vi "AlGaInPAs_prep_run_cont_dil_v15.vi"(2 "Debug Mode":bool, 3 "Elapsed Time(s)":dbl, 4 "State":enum16{"Edit", "Start", "Run", "End", "Idle"}(ring), 5 "Argument List In":string[](array[string])) -> (0 "Status Out":string, 1 "Argument List Out":string[](array[string]))   [LabVIEW 2011]
panel:
  out "Ga calculated var":u16(ring)=1 items=["Ga flow", "MFC1", "MFC2", "MFC3"]
  out "GAMFC3 var":dbl=100.0 caption="R3 (0-1000 sscm)" format="%.1f"
  out "GAMFC2 var":dbl=10.0 caption="R2 (0-100 sscm)" format="%.2f"
  out "GAMFC1 var":dbl=1.0 caption="R1 (0-10 sscm)" format="%.2f"
  out "Ga Flow var":dbl=1.0 caption="Ga Flow (0-10 sscm)" format="%.4f"
  out "Prep-In var":bool
  out "Prep-Ga var":bool
  out "Prep-Al var":bool
  out "Prep-P var":bool
  out "Prep-As var":bool
  out "prep_done":bool
  out "run started":bool
  out "first":bool=TRUE
  out "total time":dbl
  out "is OK?":bool
  out "AsH3?":bool
  out "PH3?":bool
  out "In?":bool
  out "Ga?":bool
  out "Al?":bool
  in  "Prep As":bool caption="Pre-run"
  in  "Prep P":bool caption="Pre-run"
  in  "Prep In":bool caption="Pre-run"
  in  "prep_time":dbl caption="pre-run time (s)"
  in  "Prep Al":bool caption="Pre-run"
  in  "Run As":bool caption="Run"
  in  "AsH3 Flow":dbl caption="AsH3 Flow (0-10 sccm)" format="%.2f"
  in  "P Flow":dbl caption="P Flow (0-100 sccm)" format="%.2f"
  in  "Run P":bool caption="Run"
  in  "In Flow":dbl caption="In Flow (0-100 sscm)" format="%.2f"
  in  "Run In":bool caption="Run"
  in  "Run Al":bool caption="Run"
  in  "Al Flow":dbl caption="Al Flow (0-100 sscm)" format="%.2f"
  in  "Cancel":bool
  in  "OK":bool
  out "tTotal(s) 2":dbl
  in  "Ga Tab Control":enum32{"Page 1", "Page 2", "Page 3"}(tab)
  in  "Ga Dilution":bool caption="Dilute"
  in  "Run Ga":bool caption="Run"
  in  "Prep Ga":bool caption="Pre-run"
  out "Ga Flow val":dbl=1.0 caption="Ga Flow (0-10 sscm)" format="%.4f"
  in  "Ga Flow set":dbl=1.0 caption="Ga Flow (0-10 sscm)" format="%.4f"
  out "GAMFC1 val":dbl=1.0 caption="R1 (0-10 sscm)" format="%.2f"
  out "GAMFC3 val":dbl=100.0 caption="R3 (0-1000 sscm)" format="%.1f"
  out "GAMFC2 val":dbl=10.0 caption="R2 (0-100 sscm)" format="%.2f"
  in  "GAMFC1 set":dbl=1.0 caption="R1 (0-10 sscm)" format="%.2f"
  in  "GAMFC2 set":dbl=10.0 caption="R2 (0-100 sscm)" format="%.2f"
  in  "GAMFC3 set":dbl=100.0 caption="R3 (0-1000 sscm)" format="%.1f"
  in  "Ga calculated":u16(ring)=1 items=["Ga flow", "MFC1", "MFC2", "MFC3"]
  # "Add pre-run time to run time in editor."
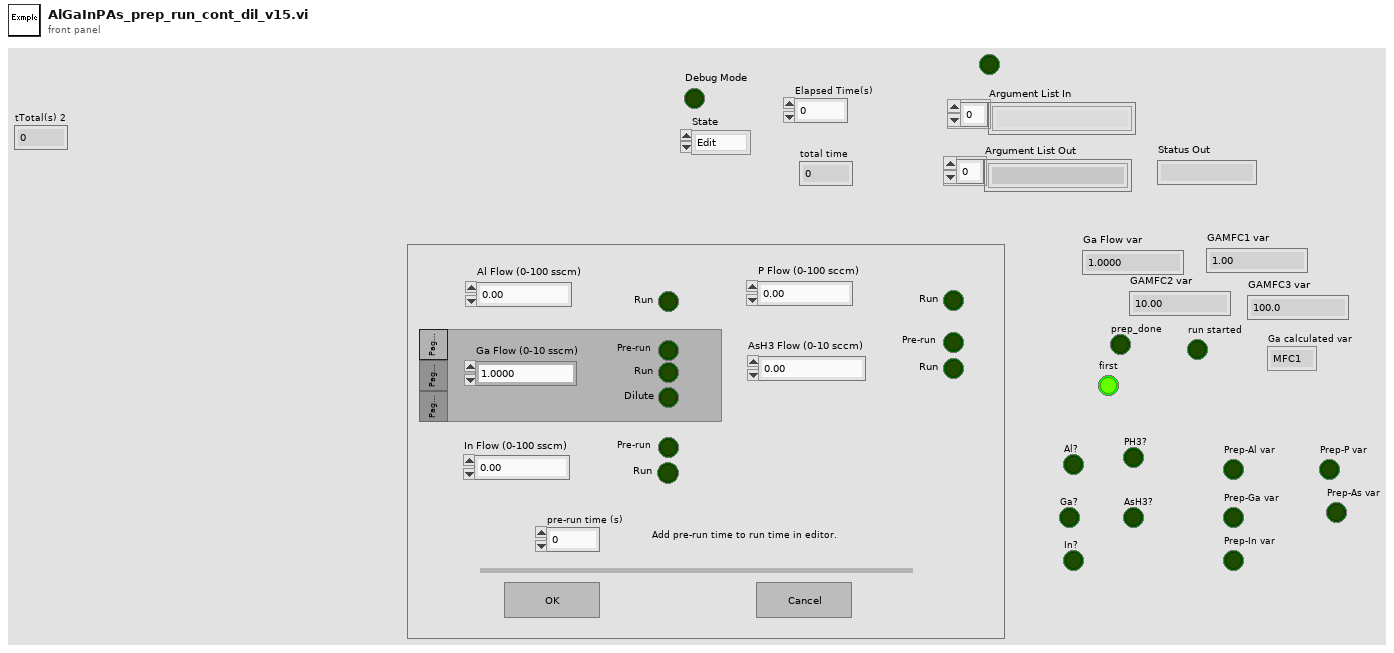
[diagram p1: front panel]
types:
  T1 = enum16{"Discrete", "Continuous", "Instantaneous", "Finite"}
  T2 = enum32{"Invalid", "Default", "Floating", "Floating/Auto-Hide", "Modal"}
  T3 = cluster{"Visible":bool, "Visible":bool, "Visible":bool, "Visible":bool, "Visible":bool, "Visible":bool, "Visible":bool, "Visible":bool}
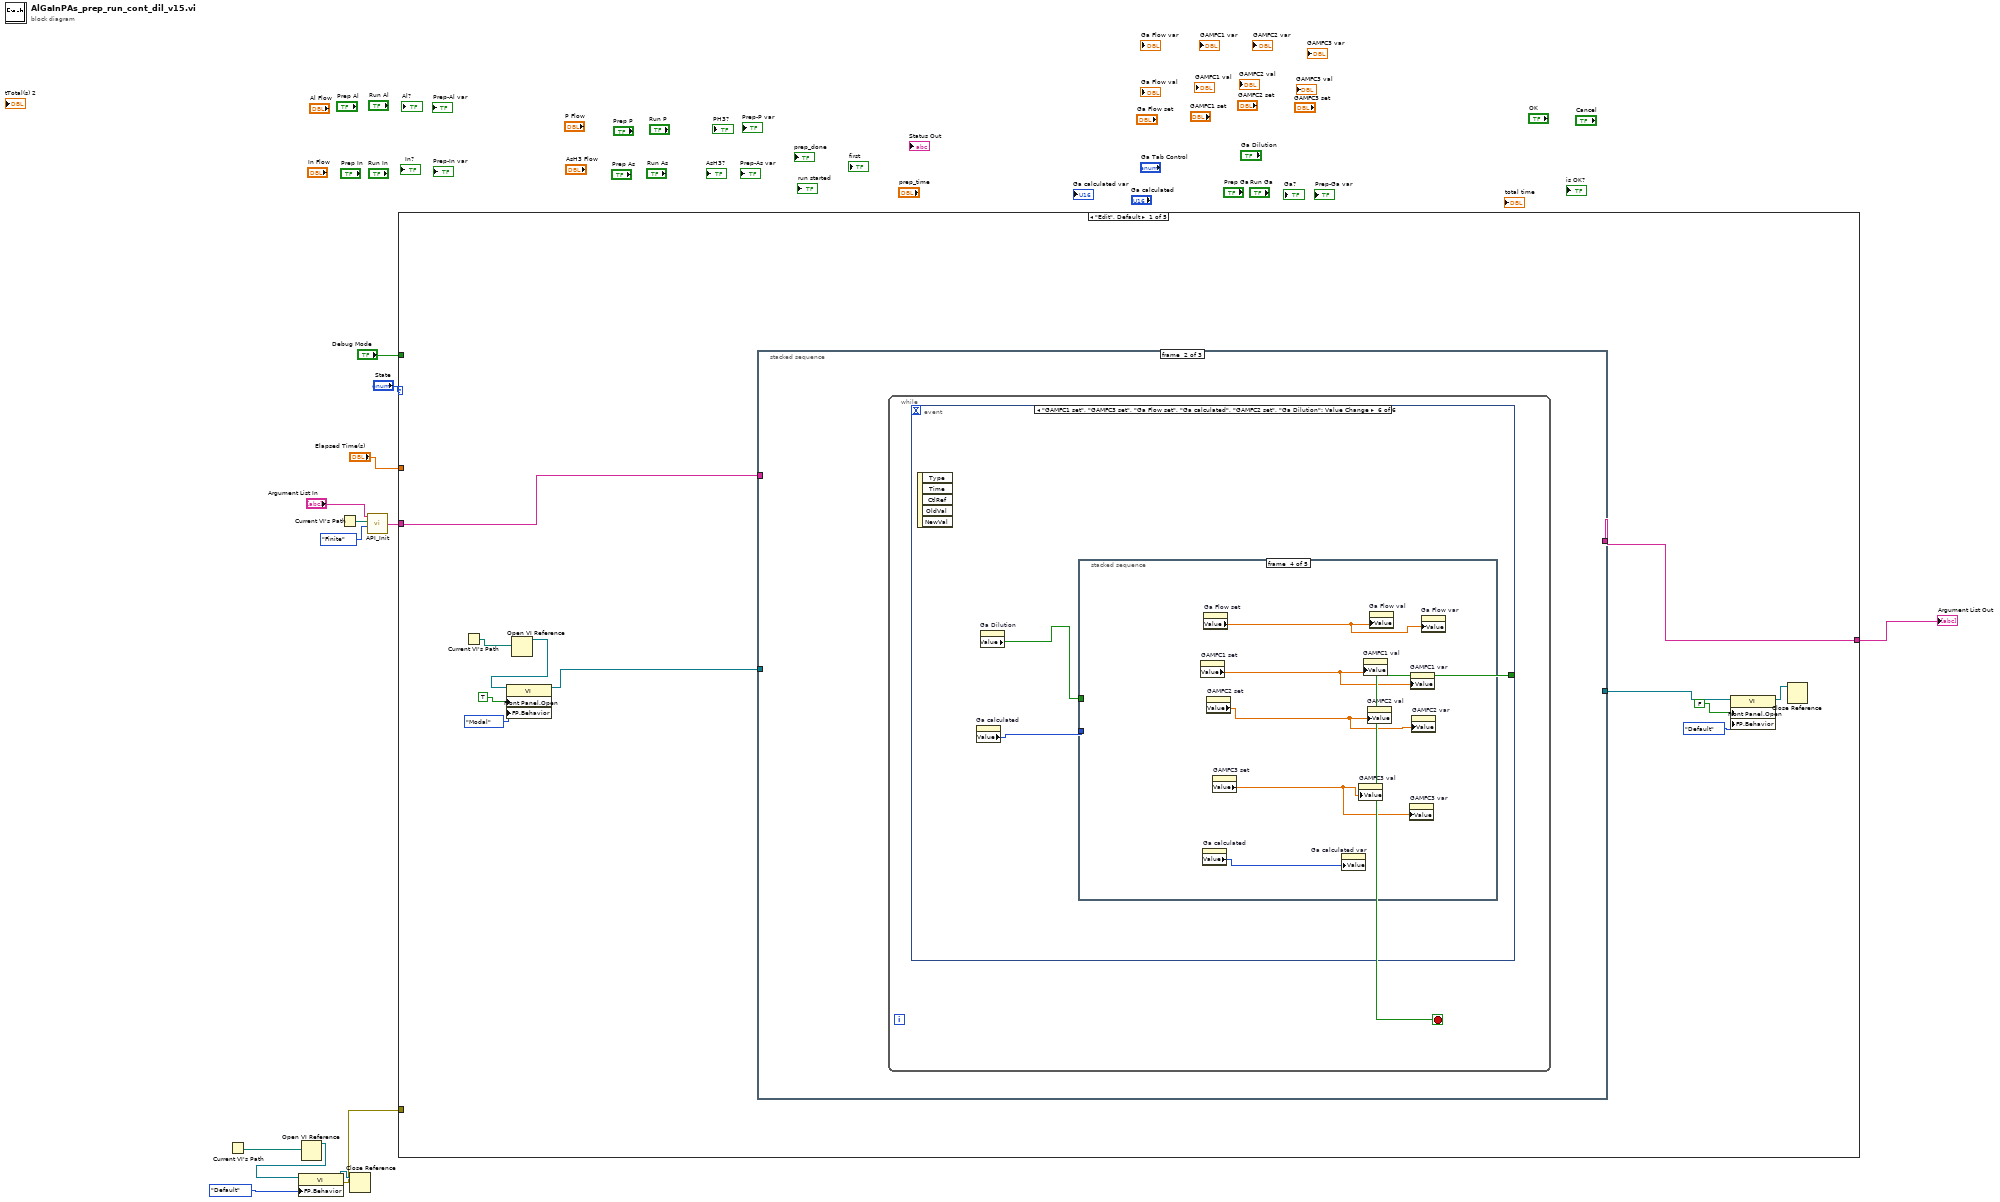
[diagram p0: block diagram]
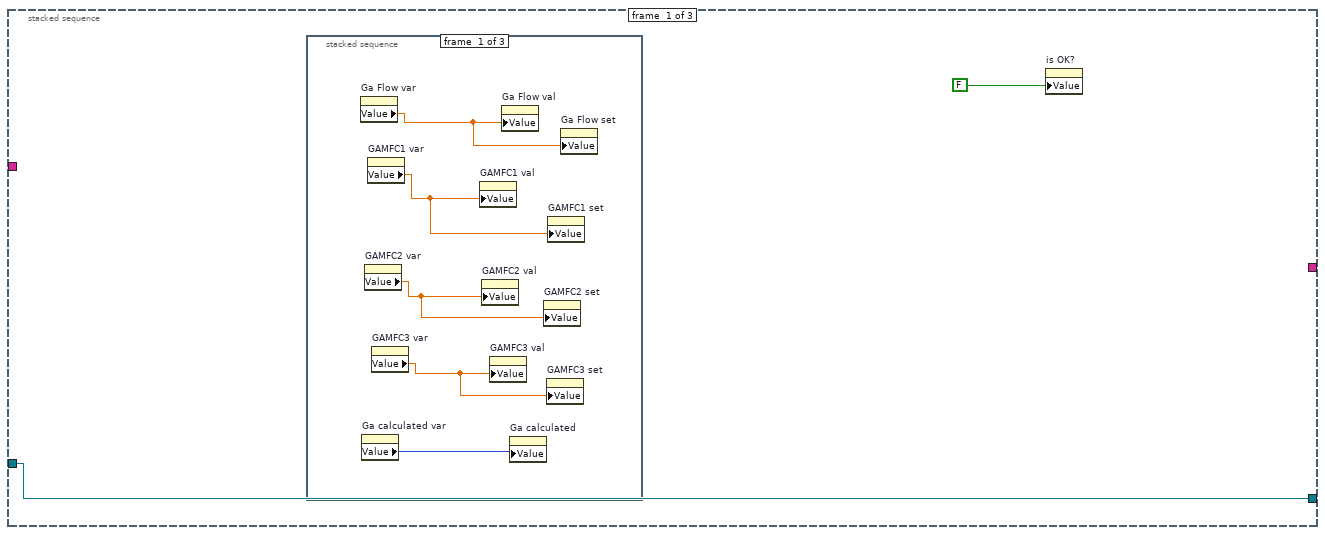
[diagram p2: hidden frame]
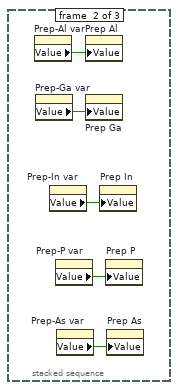
[diagram p3: hidden frame]
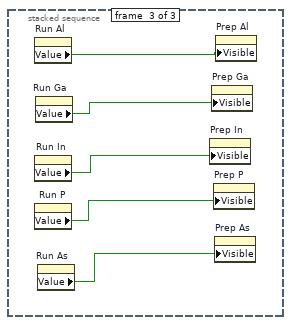
[diagram p4: hidden frame]
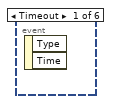
[diagram p5: hidden frame]
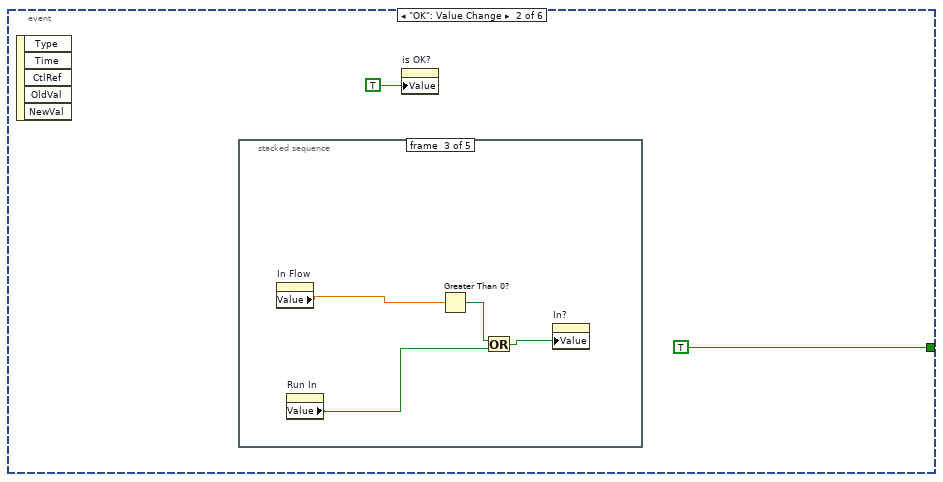
[diagram p6: hidden frame]
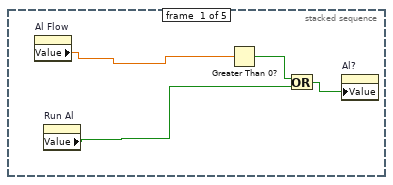
[diagram p7: hidden frame]
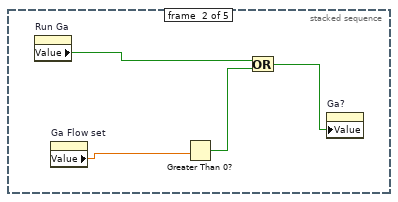
[diagram p8: hidden frame]
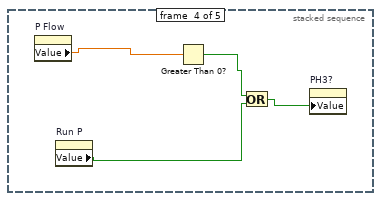
[diagram p9: hidden frame]
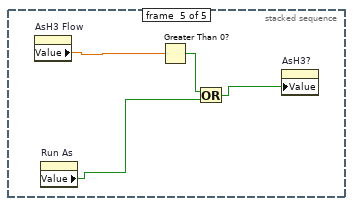
[diagram p10: hidden frame]
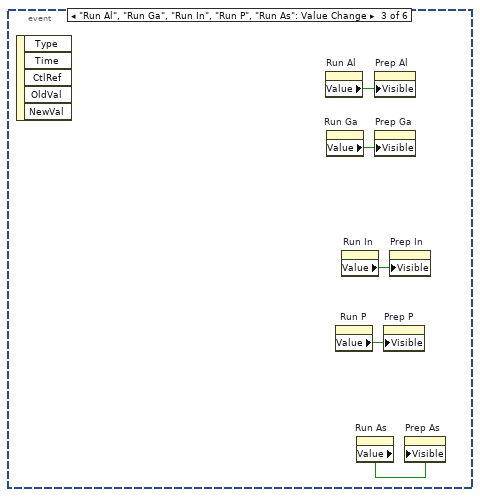
[diagram p11: hidden frame]
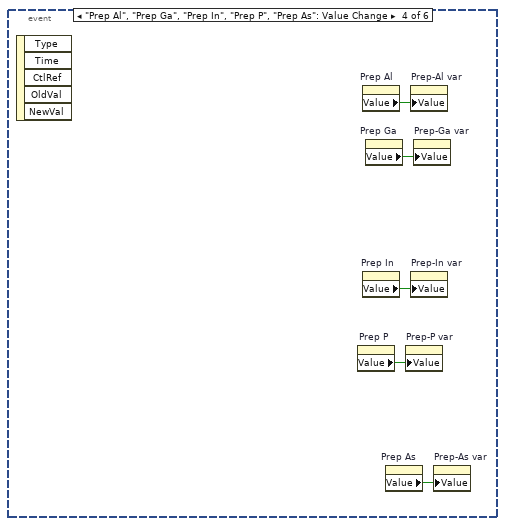
[diagram p12: hidden frame]
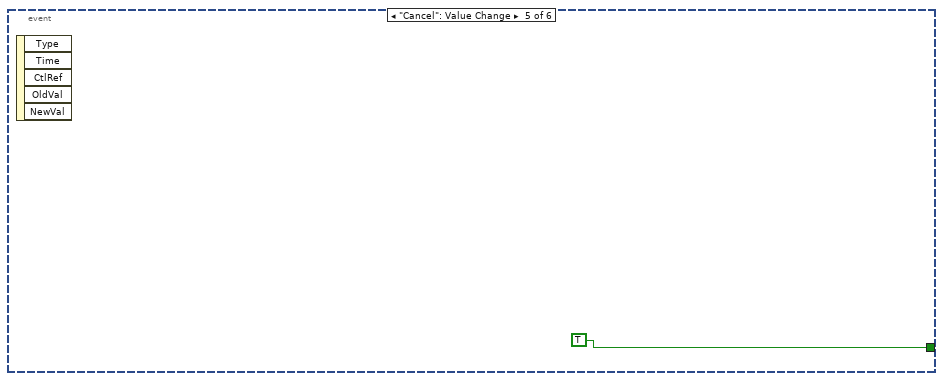
[diagram p13: hidden frame]
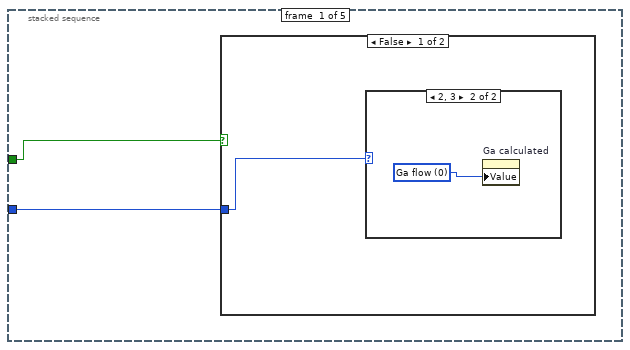
[diagram p14: hidden frame]
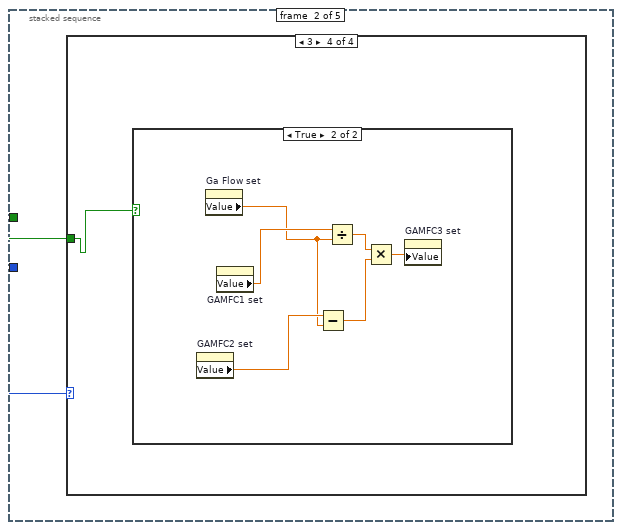
[diagram p17: hidden frame]
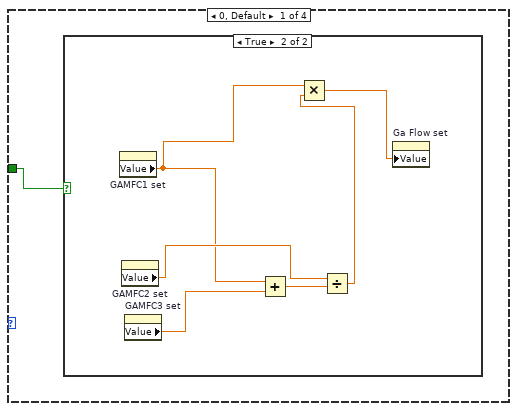
[diagram p18: hidden frame]
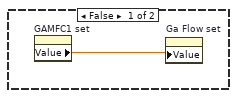
[diagram p19: hidden frame]
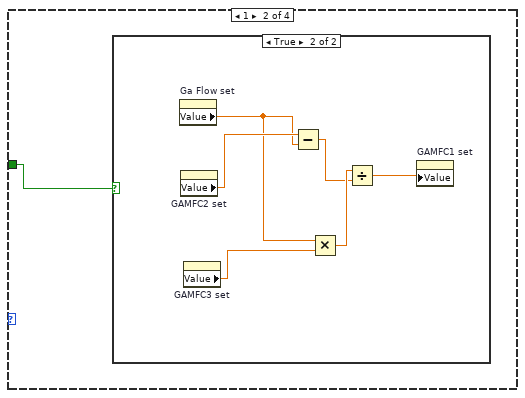
[diagram p20: hidden frame]
diagram:
  n1 = Current VI's Path() -> (path=w9:path)
  n2 = Open VI Reference(vi path=w9) -> (vi reference=w8:refnum<vi>)  [unwired: 1 in, 5 out]
  n3 = property class="VI"(reference=w8, "FP.Behavior"=T2."Default" ("Front Panel Window:Behavior")) -> (reference out=w6:refnum<vi>, error out=w5:errorcluster)  [unwired: 1 in]
  n4 = Current VI's Path() -> (path=w4:path)
  n5 = Close Reference(reference=w6) -> ()  [unwired: 1 in, 1 out]
  n6 = call "API_Init.vi"("API Mode"=T1."Finite", "VI Path"=w4, "Argument List In"="Argument List In") -> ("Argument List Out"=w1:string[])  [unwired: 1 in]
  n7 = case shown="\"Edit\", Default" "State" {
    tunnel: "Debug Mode" -> [_ w175 w229 _ _]
    tunnel: "Elapsed Time(s)" -> [_ _ w231 _ _]
    tunnel: w1 -> [w15 w177 w228 w346 w347]
    tunnel: [w14 w176 w230 w346 w347] -> w10
    tunnel: w5 -> [_ _ _ _ _]
    frame "Edit", Default {
      n8 = Current VI's Path() -> (path=w20:path)
      n9 = Open VI Reference(vi path=w20) -> (vi reference=w19:refnum<vi>)  [unwired: 1 in, 5 out]
      n10 = property class="VI"(reference=w19, "Front Panel.Open"=TRUE ("Front Panel Window:Open"), "FP.Behavior"=T2."Modal" ("Front Panel Window:Behavior")) -> (reference out=w18:refnum<vi>)  [unwired: 1 in, 1 out]
      n11 = stacked-sequence {
        tunnel: w15 -> [_ _ w170]
        tunnel: w18 -> [w26 _ _]
        tunnel: [w26 _ _] -> w22
        tunnel: [_ _ w168] -> w14
        frame #0 {
          n12 = stacked-sequence {
            frame #0 {
              n13 = property on="Ga Flow var" class="DigNum (strict)"() -> ("Value"=w31:dbl)  [unwired: 2 in, 2 out]
              n14 = property on="Ga calculated var" class="Ring (strict)"() -> ("Value"=w27:u16)  [unwired: 2 in, 2 out]
              n15 = property on="GAMFC2 var" class="DigNum (strict)"() -> ("Value"=w29:dbl)  [unwired: 2 in, 2 out]
              n16 = property on="GAMFC1 var" class="DigNum (strict)"() -> ("Value"=w28:dbl)  [unwired: 2 in, 2 out]
              n17 = property on="GAMFC3 var" class="DigNum (strict)"() -> ("Value"=w30:dbl)  [unwired: 2 in, 2 out]
              n18 = property on="GAMFC1 val" class="DigNum (strict)"("Value"=w28) -> ()  [unwired: 2 in, 2 out]
              n19 = property on="GAMFC2 val" class="DigNum (strict)"("Value"=w29) -> ()  [unwired: 2 in, 2 out]
              n20 = property on="GAMFC3 val" class="DigNum (strict)"("Value"=w30) -> ()  [unwired: 2 in, 2 out]
              n21 = property on="Ga Flow val" class="DigNum (strict)"("Value"=w31) -> ()  [unwired: 2 in, 2 out]
              n22 = property on="Ga calculated" class="Ring (strict)"("Value"=w27) -> ()  [unwired: 2 in, 2 out]
              n23 = property on="GAMFC2 set" class="DigNum (strict)"("Value"=w29) -> ()  [unwired: 2 in, 2 out]
              n24 = property on="GAMFC3 set" class="DigNum (strict)"("Value"=w30) -> ()  [unwired: 2 in, 2 out]
              n25 = property on="GAMFC1 set" class="DigNum (strict)"("Value"=w28) -> ()  [unwired: 2 in, 2 out]
              n26 = property on="Ga Flow set" class="DigNum (strict)"("Value"=w31) -> ()  [unwired: 2 in, 2 out]
            }
            frame #1 {
              n27 = property on="Prep-Al var" class="Bool (strict)"() -> ("Value"=w36:bool)  [unwired: 2 in, 2 out]
              n28 = property on="Prep-Ga var" class="Bool (strict)"() -> ("Value"=w35:bool)  [unwired: 2 in, 2 out]
              n29 = property on="Prep-In var" class="Bool (strict)"() -> ("Value"=w34:bool)  [unwired: 2 in, 2 out]
              n30 = property on="Prep-P var" class="Bool (strict)"() -> ("Value"=w33:bool)  [unwired: 2 in, 2 out]
              n31 = property on="Prep-As var" class="Bool (strict)"() -> ("Value"=w32:bool)  [unwired: 2 in, 2 out]
              n32 = property on="Prep Al" class="Bool (strict)"("Value"=w36) -> ()  [unwired: 2 in, 2 out]
              n33 = property on="Prep Ga" class="Bool (strict)"("Value"=w35) -> ()  [unwired: 2 in, 2 out]
              n34 = property on="Prep In" class="Bool (strict)"("Value"=w34) -> ()  [unwired: 2 in, 2 out]
              n35 = property on="Prep P" class="Bool (strict)"("Value"=w33) -> ()  [unwired: 2 in, 2 out]
              n36 = property on="Prep As" class="Bool (strict)"("Value"=w32) -> ()  [unwired: 2 in, 2 out]
            }
            frame #2 {
              n37 = property on="Run Al" class="Bool (strict)"() -> ("Value"=w41:bool)  [unwired: 2 in, 2 out]
              n38 = property on="Run In" class="Bool (strict)"() -> ("Value"=w39:bool)  [unwired: 2 in, 2 out]
              n39 = property on="Run P" class="Bool (strict)"() -> ("Value"=w38:bool)  [unwired: 2 in, 2 out]
              n40 = property on="Run Ga" class="Bool (strict)"() -> ("Value"=w40:bool)  [unwired: 2 in, 2 out]
              n41 = property on="Run As" class="Bool (strict)"() -> ("Value"=w37:bool)  [unwired: 2 in, 2 out]
              n42 = property on="Prep In" class="Bool (strict)"("Visible"=w39) -> ()  [unwired: 2 in, 2 out]
              n43 = property on="Prep Ga" class="Bool (strict)"("Visible"=w40) -> ()  [unwired: 2 in, 2 out]
              n44 = property on="Prep P" class="Bool (strict)"("Visible"=w38) -> ()  [unwired: 2 in, 2 out]
              n45 = property on="Prep As" class="Bool (strict)"("Visible"=w37) -> ()  [unwired: 2 in, 2 out]
              n46 = property on="Prep Al" class="Bool (strict)"("Visible"=w41) -> ()  [unwired: 2 in, 2 out]
            }
          }
          n47 = property on="is OK?" class="Bool (strict)"("Value"=FALSE ("is OK?")) -> ()  [unwired: 2 in, 2 out]
        }
        frame #1 {
          n48 = while {
            stop <- w42 stop-if-true
            n49 = event shown="[5] \"GAMFC1 set\", \"GAMFC3 set\", \"Ga Flow set\", \"Ga calculated\", \"GAMFC2 set\", \"Ga Dilution\": Value Change" {
              selector: _ -> [_ _ _ _ _ _]
              dyn-events: _ -> [_ _ _ _ _ _]
              timeout: _ -> [_ _ _ _ _ _]
              tunnel: [_ TRUE _ _ TRUE _] -> w42
              event Timeout {
                n50 = event-data() -> ()  [unwired: 1 in, 2 out]
              }
              event "OK": Value Change {
                n51 = event-data() -> ()  [unwired: 1 in, 5 out]
                n52 = stacked-sequence {
                  frame #0 {
                    n53 = property on="Al Flow" class="DigNum (strict)"() -> ("Value"=w47:dbl)  [unwired: 2 in, 2 out]
                    n54 = property on="Run Al" class="Bool (strict)"() -> ("Value"=w46:bool)  [unwired: 2 in, 2 out]
                    n55 = Greater Than 0?(x=w47) -> (x > 0?=w48:bool)
                    n56 = Or(x=w48, y=w46) -> (x .or. y?=w45:bool)
                    n57 = property on="Al?" class="Bool (strict)"("Value"=w45) -> ()  [unwired: 2 in, 2 out]
                  }
                  frame #1 {
                    n58 = property on="Run Ga" class="Bool (strict)"() -> ("Value"=w50:bool)  [unwired: 2 in, 2 out]
                    n59 = property on="Ga Flow set" class="DigNum (strict)"() -> ("Value"=w51:dbl)  [unwired: 2 in, 2 out]
                    n60 = Greater Than 0?(x=w51) -> (x > 0?=w52:bool)
                    n61 = Or(x=w50, y=w52) -> (x .or. y?=w49:bool)
                    n62 = property on="Ga?" class="Bool (strict)"("Value"=w49) -> ()  [unwired: 2 in, 2 out]
                  }
                  frame #2 {
                    n63 = property on="In Flow" class="DigNum (strict)"() -> ("Value"=w54:dbl)  [unwired: 2 in, 2 out]
                    n64 = property on="Run In" class="Bool (strict)"() -> ("Value"=w55:bool)  [unwired: 2 in, 2 out]
                    n65 = Greater Than 0?(x=w54) -> (x > 0?=w56:bool)
                    n66 = Or(x=w56, y=w55) -> (x .or. y?=w53:bool)
                    n67 = property on="In?" class="Bool (strict)"("Value"=w53) -> ()  [unwired: 2 in, 2 out]
                  }
                  frame #3 {
                    n68 = property on="P Flow" class="DigNum (strict)"() -> ("Value"=w59:dbl)  [unwired: 2 in, 2 out]
                    n69 = property on="Run P" class="Bool (strict)"() -> ("Value"=w58:bool)  [unwired: 2 in, 2 out]
                    n70 = Greater Than 0?(x=w59) -> (x > 0?=w60:bool)
                    n71 = Or(x=w60, y=w58) -> (x .or. y?=w57:bool)
                    n72 = property on="PH3?" class="Bool (strict)"("Value"=w57) -> ()  [unwired: 2 in, 2 out]
                  }
                  frame #4 {
                    n73 = property on="AsH3 Flow" class="DigNum (strict)"() -> ("Value"=w63:dbl)  [unwired: 2 in, 2 out]
                    n74 = property on="Run As" class="Bool (strict)"() -> ("Value"=w62:bool)  [unwired: 2 in, 2 out]
                    n75 = Greater Than 0?(x=w63) -> (x > 0?=w64:bool)
                    n76 = Or(x=w64, y=w62) -> (x .or. y?=w61:bool)
                    n77 = property on="AsH3?" class="Bool (strict)"("Value"=w61) -> ()  [unwired: 2 in, 2 out]
                  }
                }
                n78 = property on="is OK?" class="Bool (strict)"("Value"=TRUE ("is OK?")) -> ()  [unwired: 2 in, 2 out]
              }
              event "Run Al", "Run Ga", "Run In", "Run P", "Run As": Value Change {
                n79 = event-data() -> ()  [unwired: 1 in, 5 out]
                n80 = property on="Run Al" class="Bool (strict)"() -> ("Value"=w69:bool)  [unwired: 2 in, 2 out]
                n81 = property on="Run Ga" class="Bool (strict)"() -> ("Value"=w68:bool)  [unwired: 2 in, 2 out]
                n82 = property on="Run P" class="Bool (strict)"() -> ("Value"=w65:bool)  [unwired: 2 in, 2 out]
                n83 = property on="Run In" class="Bool (strict)"() -> ("Value"=w67:bool)  [unwired: 2 in, 2 out]
                n84 = property on="Run As" class="Bool (strict)"() -> ("Value"=w66:bool)  [unwired: 2 in, 2 out]
                n85 = property on="Prep Al" class="Bool (strict)"("Visible"=w69) -> ()  [unwired: 2 in, 2 out]
                n86 = property on="Prep Ga" class="Bool (strict)"("Visible"=w68) -> ()  [unwired: 2 in, 2 out]
                n87 = property on="Prep P" class="Bool (strict)"("Visible"=w65) -> ()  [unwired: 2 in, 2 out]
                n88 = property on="Prep In" class="Bool (strict)"("Visible"=w67) -> ()  [unwired: 2 in, 2 out]
                n89 = property on="Prep As" class="Bool (strict)"("Visible"=w66) -> ()  [unwired: 2 in, 2 out]
              }
              event "Prep Al", "Prep Ga", "Prep In", "Prep P", "Prep As": Value Change {
                n90 = event-data() -> ()  [unwired: 1 in, 5 out]
                n91 = property on="Prep P" class="Bool (strict)"() -> ("Value"=w71:bool)  [unwired: 2 in, 2 out]
                n92 = property on="Prep Al" class="Bool (strict)"() -> ("Value"=w74:bool)  [unwired: 2 in, 2 out]
                n93 = property on="Prep In" class="Bool (strict)"() -> ("Value"=w72:bool)  [unwired: 2 in, 2 out]
                n94 = property on="Prep Ga" class="Bool (strict)"() -> ("Value"=w73:bool)  [unwired: 2 in, 2 out]
                n95 = property on="Prep As" class="Bool (strict)"() -> ("Value"=w70:bool)  [unwired: 2 in, 2 out]
                n96 = property on="Prep-P var" class="Bool (strict)"("Value"=w71) -> ()  [unwired: 2 in, 2 out]
                n97 = property on="Prep-Al var" class="Bool (strict)"("Value"=w74) -> ()  [unwired: 2 in, 2 out]
                n98 = property on="Prep-In var" class="Bool (strict)"("Value"=w72) -> ()  [unwired: 2 in, 2 out]
                n99 = property on="Prep-Ga var" class="Bool (strict)"("Value"=w73) -> ()  [unwired: 2 in, 2 out]
                n100 = property on="Prep-As var" class="Bool (strict)"("Value"=w70) -> ()  [unwired: 2 in, 2 out]
              }
              event "Cancel": Value Change {
                n101 = event-data() -> ()  [unwired: 1 in, 5 out]
              }
              event "GAMFC1 set", "GAMFC3 set", "Ga Flow set", "Ga calculated", "GAMFC2 set", "Ga Dilution": Value Change {
                n102 = event-data() -> ()  [unwired: 1 in, 5 out]
                n103 = property on="Ga calculated" class="Ring (strict)"() -> ("Value"=w76:u16)  [unwired: 2 in, 2 out]
                n104 = property on="Ga Dilution" class="Bool (strict)"() -> ("Value"=w77:bool)  [unwired: 2 in, 2 out]
                n105 = stacked-sequence {
                  tunnel: w77 -> [w78 w83 w124 _ w164]
                  tunnel: w76 -> [w79 w82 w123 _ _]
                  frame #0 {
                    n106 = case shown="False" w78 {
                      tunnel: w79 -> [w80 _]
                      frame False {
                        n107 = case shown="2, 3" w80 {
                          frame 0, 1, Default {
                          }
                          frame 2, 3 {
                            w81 = u16 0 items=["Ga flow", "MFC1", "MFC2", "MFC3"] ("Ga calculated")
                            n108 = property on="Ga calculated" class="Ring (strict)"("Value"=w81) -> ()  [unwired: 2 in, 2 out]
                          }
                        }
                      }
                      frame True {
                      }
                    }
                  }
                  frame #1 {
                    n109 = case shown="3" w82 {
                      tunnel: w83 -> [w84 w92 w100 w107]
                      frame 0, Default {
                        n110 = case shown="True" w84 {
                          frame False {
                            n111 = property on="GAMFC1 set" class="DigNum (strict)"() -> ("Value"=w85:dbl)  [unwired: 2 in, 2 out]
                            n112 = property on="Ga Flow set" class="DigNum (strict)"("Value"=w85) -> ()  [unwired: 2 in, 2 out]
                          }
                          frame True {
                            n113 = property on="GAMFC1 set" class="DigNum (strict)"() -> ("Value"=w87:dbl)  [unwired: 2 in, 2 out]
                            n114 = property on="GAMFC2 set" class="DigNum (strict)"() -> ("Value"=w89:dbl)  [unwired: 2 in, 2 out]
                            n115 = property on="GAMFC3 set" class="DigNum (strict)"() -> ("Value"=w91:dbl)  [unwired: 2 in, 2 out]
                            n116 = Add(x=w87, y=w91) -> (x+y=w90:dbl)
                            n117 = Divide(x=w89, y=w90) -> (x/y=w88:dbl)
                            n118 = Multiply(x=w87, y=w88) -> (x*y=w86:dbl)
                            n119 = property on="Ga Flow set" class="DigNum (strict)"("Value"=w86) -> ()  [unwired: 2 in, 2 out]
                          }
                        }
                      }
                      frame 1 {
                        n120 = case shown="True" w92 {
                          frame False {
                            n121 = property on="Ga Flow set" class="DigNum (strict)"() -> ("Value"=w93:dbl)  [unwired: 2 in, 2 out]
                            n122 = property on="GAMFC1 set" class="DigNum (strict)"("Value"=w93) -> ()  [unwired: 2 in, 2 out]
                          }
                          frame True {
                            n123 = property on="Ga Flow set" class="DigNum (strict)"() -> ("Value"=w98:dbl)  [unwired: 2 in, 2 out]
                            n124 = property on="GAMFC2 set" class="DigNum (strict)"() -> ("Value"=w99:dbl)  [unwired: 2 in, 2 out]
                            n125 = property on="GAMFC3 set" class="DigNum (strict)"() -> ("Value"=w97:dbl)  [unwired: 2 in, 2 out]
                            n126 = Subtract(x=w99, y=w98) -> (x-y=w95:dbl)
                            n127 = Multiply(x=w98, y=w97) -> (x*y=w96:dbl)
                            n128 = Divide(x=w96, y=w95) -> (x/y=w94:dbl)
                            n129 = property on="GAMFC1 set" class="DigNum (strict)"("Value"=w94) -> ()  [unwired: 2 in, 2 out]
                          }
                        }
                      }
                      frame 2 {
                        n130 = case shown="True" w100 {
                          frame False {
                          }
                          frame True {
                            n131 = property on="GAMFC1 set" class="DigNum (strict)"() -> ("Value"=w102:dbl)  [unwired: 2 in, 2 out]
                            n132 = property on="GAMFC3 set" class="DigNum (strict)"() -> ("Value"=w104:dbl)  [unwired: 2 in, 2 out]
                            n133 = property on="Ga Flow set" class="DigNum (strict)"() -> ("Value"=w105:dbl)  [unwired: 2 in, 2 out]
                            n134 = Add(x=w102, y=w104) -> (x+y=w106:dbl)
                            n135 = Multiply(x=w105, y=w106) -> (x*y=w103:dbl)
                            n136 = Divide(x=w103, y=w102) -> (x/y=w101:dbl)
                            n137 = property on="GAMFC2 set" class="DigNum (strict)"("Value"=w101) -> ()  [unwired: 2 in, 2 out]
                          }
                        }
                      }
                      frame 3 {
                        n138 = case shown="True" w107 {
                          frame False {
                          }
                          frame True {
                            n139 = property on="GAMFC2 set" class="DigNum (strict)"() -> ("Value"=w113:dbl)  [unwired: 2 in, 2 out]
                            n140 = property on="Ga Flow set" class="DigNum (strict)"() -> ("Value"=w111:dbl)  [unwired: 2 in, 2 out]
                            n141 = property on="GAMFC1 set" class="DigNum (strict)"() -> ("Value"=w112:dbl)  [unwired: 2 in, 2 out]
                            n142 = Subtract(x=w113, y=w111) -> (x-y=w109:dbl)
                            n143 = Divide(x=w112, y=w111) -> (x/y=w110:dbl)
                            n144 = Multiply(x=w110, y=w109) -> (x*y=w108:dbl)
                            n145 = property on="GAMFC3 set" class="DigNum (strict)"("Value"=w108) -> ()  [unwired: 2 in, 2 out]
                          }
                        }
                      }
                    }
                  }
                  frame #2 {
                    n146 = case shown="3" w123 {
                      tunnel: w124 -> [w125 w134 w141 w151]
                      tunnel: [w126 w133 w142 w150] -> w122
                      frame 0, Default {
                        n147 = case shown="False" w125 {
                          tunnel: [w127 w132] -> w126
                          frame False {
                            w128 = TRUE ("Visible")
                            w129 = FALSE ("Visible")
                            n148 = Bundle("Visible"=w129, "Visible"=w128, "Visible"=w129, "Visible"=w129, "Visible"=w128, "Visible"=w129, "Visible"=w129, "Visible"=w129) -> (w127:T3)  [unwired: 1 in]
                          }
                          frame True {
                            w130 = TRUE ("Visible")
                            w131 = FALSE ("Visible")
                            n149 = Bundle("Visible"=w131, "Visible"=w130, "Visible"=w130, "Visible"=w130, "Visible"=w130, "Visible"=w131, "Visible"=w131, "Visible"=w131) -> (w132:T3)  [unwired: 1 in]
                          }
                        }
                      }
                      frame 1 {
                        n150 = case shown="False" w134 {
                          tunnel: [w137 w138] -> w133
                          frame False {
                            w135 = TRUE ("Visible")
                            w136 = FALSE ("Visible")
                            n151 = Bundle("Visible"=w135, "Visible"=w136, "Visible"=w136, "Visible"=w136, "Visible"=w136, "Visible"=w135, "Visible"=w136, "Visible"=w136) -> (w137:T3)  [unwired: 1 in]
                          }
                          frame True {
                            w140 = TRUE ("Visible")
                            w139 = FALSE ("Visible")
                            n152 = Bundle("Visible"=w140, "Visible"=w139, "Visible"=w140, "Visible"=w140, "Visible"=w139, "Visible"=w140, "Visible"=w139, "Visible"=w139) -> (w138:T3)  [unwired: 1 in]
                          }
                        }
                      }
                      frame 2 {
                        n153 = case shown="False" w141 {
                          tunnel: [w146 w147] -> w142
                          frame False {
                            w145 = u16 1 items=["Ga flow", "MFC1", "MFC2", "MFC3"] ("Ga calculated")
                            w144 = TRUE ("Visible")
                            w143 = FALSE ("Visible")
                            n154 = property on="Ga calculated" class="Ring (strict)"("Value"=w145) -> ()  [unwired: 2 in, 2 out]
                            n155 = Bundle("Visible"=w144, "Visible"=w144, "Visible"=w143, "Visible"=w143, "Visible"=w143, "Visible"=w144, "Visible"=w143, "Visible"=w143) -> (w146:T3)  [unwired: 1 in]
                          }
                          frame True {
                            w149 = TRUE ("Visible")
                            w148 = FALSE ("Visible")
                            n156 = Bundle("Visible"=w149, "Visible"=w149, "Visible"=w148, "Visible"=w149, "Visible"=w148, "Visible"=w148, "Visible"=w149, "Visible"=w148) -> (w147:T3)  [unwired: 1 in]
                          }
                        }
                      }
                      frame 3 {
                        n157 = case shown="False" w151 {
                          tunnel: [w155 w158] -> w150
                          frame False {
                            w154 = u16 1 items=["Ga flow", "MFC1", "MFC2", "MFC3"] ("Ga calculated")
                            w153 = TRUE ("Visible")
                            w152 = FALSE ("Visible")
                            n158 = property on="Ga calculated" class="Ring (strict)"("Value"=w154) -> ()  [unwired: 2 in, 2 out]
                            n159 = Bundle("Visible"=w153, "Visible"=w153, "Visible"=w152, "Visible"=w152, "Visible"=w152, "Visible"=w153, "Visible"=w152, "Visible"=w152) -> (w155:T3)  [unwired: 1 in]
                          }
                          frame True {
                            w157 = TRUE ("Visible")
                            w156 = FALSE ("Visible")
                            n160 = Bundle("Visible"=w157, "Visible"=w157, "Visible"=w157, "Visible"=w156, "Visible"=w156, "Visible"=w156, "Visible"=w156, "Visible"=w157) -> (w158:T3)  [unwired: 1 in]
                          }
                        }
                      }
                    }
                    n161 = Unbundle(w122) -> ("Visible"=w121:bool, "Visible"=w120:bool, "Visible"=w119:bool, "Visible"=w118:bool, "Visible"=w117:bool, "Visible"=w116:bool, "Visible"=w115:bool, "Visible"=w114:bool)
                    n162 = property on="Ga Flow val" class="DigNum (strict)"("Visible"=w117) -> ()  [unwired: 2 in, 2 out]
                    n163 = property on="Ga Flow set" class="DigNum (strict)"("Visible"=w121) -> ()  [unwired: 2 in, 2 out]
                    n164 = property on="GAMFC1 set" class="DigNum (strict)"("Visible"=w120) -> ()  [unwired: 2 in, 2 out]
                    n165 = property on="GAMFC3 set" class="DigNum (strict)"("Visible"=w118) -> ()  [unwired: 2 in, 2 out]
                    n166 = property on="GAMFC1 val" class="DigNum (strict)"("Visible"=w116) -> ()  [unwired: 2 in, 2 out]
                    n167 = property on="GAMFC2 set" class="DigNum (strict)"("Visible"=w119) -> ()  [unwired: 2 in, 2 out]
                    n168 = property on="GAMFC2 val" class="DigNum (strict)"("Visible"=w115) -> ()  [unwired: 2 in, 2 out]
                    n169 = property on="GAMFC3 val" class="DigNum (strict)"("Visible"=w114) -> ()  [unwired: 2 in, 2 out]
                  }
                  frame #3 {
                    n170 = property on="GAMFC1 set" class="DigNum (strict)"() -> ("Value"=w162:dbl)  [unwired: 2 in, 2 out]
                    n171 = property on="Ga calculated" class="Ring (strict)"() -> ("Value"=w159:u16)  [unwired: 2 in, 2 out]
                    n172 = property on="Ga Flow set" class="DigNum (strict)"() -> ("Value"=w163:dbl)  [unwired: 2 in, 2 out]
                    n173 = property on="GAMFC2 set" class="DigNum (strict)"() -> ("Value"=w161:dbl)  [unwired: 2 in, 2 out]
                    n174 = property on="GAMFC3 set" class="DigNum (strict)"() -> ("Value"=w160:dbl)  [unwired: 2 in, 2 out]
                    n175 = property on="Ga calculated var" class="Ring (strict)"("Value"=w159) -> ()  [unwired: 2 in, 2 out]
                    n176 = property on="GAMFC3 val" class="DigNum (strict)"("Value"=w160) -> ()  [unwired: 2 in, 2 out]
                    n177 = property on="GAMFC1 val" class="DigNum (strict)"("Value"=w162) -> ()  [unwired: 2 in, 2 out]
                    n178 = property on="GAMFC2 val" class="DigNum (strict)"("Value"=w161) -> ()  [unwired: 2 in, 2 out]
                    n179 = property on="Ga Flow val" class="DigNum (strict)"("Value"=w163) -> ()  [unwired: 2 in, 2 out]
                    n180 = property on="GAMFC3 var" class="DigNum (strict)"("Value"=w160) -> ()  [unwired: 2 in, 2 out]
                    n181 = property on="GAMFC1 var" class="DigNum (strict)"("Value"=w162) -> ()  [unwired: 2 in, 2 out]
                    n182 = property on="GAMFC2 var" class="DigNum (strict)"("Value"=w161) -> ()  [unwired: 2 in, 2 out]
                    n183 = property on="Ga Flow var" class="DigNum (strict)"("Value"=w163) -> ()  [unwired: 2 in, 2 out]
                  }
                  frame #4 {
                    n184 = case shown="False" w164 {
                      frame False {
                        n185 = property on="Ga calculated" class="Ring (strict)"("Disabled Items []"=i32[] [2, 3]) -> ()  [unwired: 2 in, 2 out]
                      }
                      frame True {
                        n186 = property on="Ga calculated" class="Ring (strict)"("Disabled Items []"=i32[] []) -> ()  [unwired: 2 in, 2 out]
                      }
                    }
                  }
                }
              }
            }
          }
        }
        frame #2 {
          n187 = property on="is OK?" class="Bool (strict)"() -> ("Value"=w167:bool)  [unwired: 2 in, 2 out]
          n188 = case shown="True" w167 {
            tunnel: w170 -> [w173 w174]
            tunnel: [w173 w174] -> w169
            frame False {
            }
            frame True {
            }
          }
          n189 = Not(x=w167) -> (.not. x?=w172:bool)
          n190 = Current VI's Path() -> (path=w171:path)
          n191 = call "API_Edit.vi"("Cancel"=w172, "OK"=w167, "VI Path"=w171, "Argument List In"=w169) -> ("Argument List Out"=w168:string[])
        }
      }
      n192 = property class="VI"(reference=w22, "Front Panel.Open"=FALSE ("Front Panel Window:Open"), "FP.Behavior"=T2."Default" ("Front Panel Window:Behavior")) -> (reference out=w23:refnum<vi>)  [unwired: 1 in, 1 out]
      n193 = Close Reference(reference=w23) -> ()  [unwired: 1 in, 1 out]
    }
    frame "Start" {
      n194 = call "Set_Argument.vi"("Enable"=FALSE, "Argument"="run_started", "Argument List In"=w177) -> ("Argument List Out"=w176:string[])
      n195 = stacked-sequence {
        tunnel: w175 -> [w180 w189 w201 w210 w219]
        frame #0 {
          n196 = case shown="False" w180 {
            frame False {
              n197 = property on="Al?" class="Bool (strict)"() -> ("Value"=w181:bool)  [unwired: 2 in, 2 out]
              n198 = case shown="True" w181 {
                frame False {
                  w182 = FALSE ("Al Active")
                  n199 = call "set_Al.vi"("Aluminum Flow"=0.0, "Al Remote"=w182, "Al Run"=w182, "Al Bubbler"=w182, "Al Active"=w182) -> ()  [unwired: 5 out]
                }
                frame True {
                  w188 = TRUE ("Al Active")
                  n200 = property on="Prep Al" class="Bool (strict)"() -> ("Value"=w186:bool)  [unwired: 2 in, 2 out]
                  n201 = property on="Run Al" class="Bool (strict)"() -> ("Value"=w185:bool)  [unwired: 2 in, 2 out]
                  n202 = property on="Al Flow" class="DigNum (strict)"() -> ("Value"=w187:dbl)  [unwired: 2 in, 2 out]
                  n203 = And(x=w186, y=w185) -> (x .and. y?=w184:bool)
                  n204 = call "set_Al.vi"("Aluminum Flow"=w187, "Al Run"=w184, "Al Bubbler"=w188, "Al Active"=w188) -> ()  [unwired: 1 in, 5 out]
                }
              }
            }
            frame True {
            }
          }
        }
        frame #1 {
          n205 = case shown="False" w189 {
            frame False {
              n206 = property on="Ga?" class="Bool (strict)"() -> ("Value"=w190:bool)  [unwired: 2 in, 2 out]
              n207 = case shown="True" w190 {
                frame False {
                  w192 = FALSE ("Ga Active")
                  w191 = 0.0 ("Ga Flow 1")
                  n208 = call "set_Ga.vi"("Ga Active"=w192, "Ga Flow 3"=w191, "Ga Flow 2"=w191, "Ga Flow 1"=w191, "Ga Bubbler"=w192, "Ga H2 Dilute"=w192, "Ga Run"=w192, "Ga Remote"=w192) -> ()  [unwired: 8 out]
                }
                frame True {
                  w196 = TRUE ("Ga Active")
                  n209 = property on="GAMFC3 var" class="DigNum (strict)"() -> ("Value"=w193:dbl)  [unwired: 2 in, 2 out]
                  n210 = property on="GAMFC2 var" class="DigNum (strict)"() -> ("Value"=w194:dbl)  [unwired: 2 in, 2 out]
                  n211 = property on="GAMFC1 var" class="DigNum (strict)"() -> ("Value"=w195:dbl)  [unwired: 2 in, 2 out]
                  n212 = property on="Prep-Ga var" class="Bool (strict)"() -> ("Value"=w197:bool)  [unwired: 2 in, 2 out]
                  n213 = property on="Run Ga" class="Bool (strict)"() -> ("Value"=w198:bool)  [unwired: 2 in, 2 out]
                  n214 = And(x=w197, y=w198) -> (x .and. y?=w200:bool)
                  n215 = property on="Ga Dilution" class="Bool (strict)"() -> ("Value"=w199:bool)  [unwired: 2 in, 2 out]
                  n216 = call "set_Ga.vi"("Ga Active"=w196, "Ga Flow 3"=w193, "Ga Flow 2"=w194, "Ga Flow 1"=w195, "Ga Bubbler"=w196, "Ga H2 Dilute"=w199, "Ga Run"=w200, "Ga Remote"=w196) -> ()  [unwired: 8 in]
                }
              }
            }
            frame True {
            }
          }
        }
        frame #2 {
          n217 = case shown="False" w201 {
            frame False {
              n218 = property on="In?" class="Bool (strict)"() -> ("Value"=w202:bool)  [unwired: 2 in, 2 out]
              n219 = case shown="True" w202 {
                frame False {
                  w204 = FALSE ("In Remote")
                  n220 = call "set_In.vi"("Indium Flow"=0.0, "In Remote"=w204, "In Run"=w204, "In Bubbler"=w204, "In Active"=w204) -> ()  [unwired: 5 out]
                }
                frame True {
                  w209 = TRUE ("In Run")
                  n221 = property on="Run In" class="Bool (strict)"() -> ("Value"=w206:bool)  [unwired: 2 in, 2 out]
                  n222 = property on="Prep In" class="Bool (strict)"() -> ("Value"=w207:bool)  [unwired: 2 in, 2 out]
                  n223 = And(x=w207, y=w206) -> (x .and. y?=w205:bool)
                  n224 = property on="In Flow" class="DigNum (strict)"() -> ("Value"=w208:dbl)  [unwired: 2 in, 2 out]
                  n225 = call "set_In.vi"("Indium Flow"=w208, "In Run"=w205, "In Bubbler"=w209, "In Active"=w209) -> ()  [unwired: 1 in, 5 out]
                }
              }
            }
            frame True {
            }
          }
        }
        frame #3 {
          n226 = case shown="False" w210 {
            frame False {
              n227 = property on="PH3?" class="Bool (strict)"() -> ("Value"=w211:bool)  [unwired: 2 in, 2 out]
              n228 = case shown="True" w211 {
                frame False {
                  w212 = FALSE ("P_Gas Active")
                  n229 = call "set_P_gas.vi"("P_Gas Active"=w212, "P_Gas Flow"=0.0, "P_Gas In"=w212, "P_Gas H2 In"=w212, "P_Gas Run"=w212, "P_Gas Remote"=w212) -> ()  [unwired: 10 out]
                }
                frame True {
                  w218 = TRUE ("P_Gas Active")
                  n230 = property on="P Flow" class="DigNum (strict)"() -> ("Value"=w217:dbl)  [unwired: 2 in, 2 out]
                  n231 = property on="Prep P" class="Bool (strict)"() -> ("Value"=w216:bool)  [unwired: 2 in, 2 out]
                  n232 = property on="Run P" class="Bool (strict)"() -> ("Value"=w215:bool)  [unwired: 2 in, 2 out]
                  n233 = And(x=w216, y=w215) -> (x .and. y?=w214:bool)
                  n234 = call "set_P_gas.vi"("P_Gas Active"=w218, "P_Gas Flow"=w217, "P_Gas In"=w218, "P_Gas Run"=w214) -> ()  [unwired: 2 in, 10 out]
                }
              }
            }
            frame True {
            }
          }
        }
        frame #4 {
          n235 = case shown="False" w219 {
            frame False {
              n236 = property on="AsH3?" class="Bool (strict)"() -> ("Value"=w220:bool)  [unwired: 2 in, 2 out]
              n237 = case shown="True" w220 {
                frame False {
                  w221 = FALSE ("As_Gas Active")
                  n238 = call "set_As_gas.vi"("As_Gas Active"=w221, "As_Gas Flow"=0.0, "As_Gas In"=w221, "As_Gas H2"=w221, "As_Gas Run"=w221, "As_Gas Remote"=w221) -> ()  [unwired: 10 in]
                }
                frame True {
                  w227 = TRUE ("As_Gas Active")
                  n239 = property on="Prep As" class="Bool (strict)"() -> ("Value"=w224:bool)  [unwired: 2 in, 2 out]
                  n240 = property on="Run As" class="Bool (strict)"() -> ("Value"=w225:bool)  [unwired: 2 in, 2 out]
                  n241 = property on="AsH3 Flow" class="DigNum (strict)"() -> ("Value"=w226:dbl)  [unwired: 2 in, 2 out]
                  n242 = And(x=w224, y=w225) -> (x .and. y?=w223:bool)
                  n243 = call "set_As_gas.vi"("As_Gas Active"=w227, "As_Gas Flow"=w226, "As_Gas In"=w227, "As_Gas Run"=w223) -> ()  [unwired: 12 in]
                }
              }
            }
            frame True {
            }
          }
        }
      }
    }
    frame "Run" {
      n244 = stacked-sequence {
        tunnel: w231 -> [_ w236 _ _]
        tunnel: w228 -> [w233 _ _ w290]
        tunnel: [_ _ _ w289] -> w230
        tunnel: w229 -> [_ _ _ w291]
        frame #0 {
          n245 = call "Get_Argument.vi"("Argument"="run_started", "Argument List"=w233) -> ("Enabled"=w232:bool)
          n246 = local write "run started"(w232) -> ()
        }
        frame #1 {
          n247 = property on="prep_time" class="DigNum (strict)"() -> ("Value"=w237:dbl)  [unwired: 2 in, 2 out]
          n248 = Greater Or Equal?(x=w236, y=w237) -> (x >= y?=w235:bool)
          n249 = local write "prep_done"(w235) -> ()
        }
        frame #2 {
          n250 = local read "run started"() -> (w239:bool)
          n251 = Not(x=w239) -> (.not. x?=w238:bool)
          n252 = stacked-sequence {
            tunnel: w238 -> [w241 w245 w254 w263 w272 w281]
            frame #0 {
              n253 = case shown="True" w241 {
                tunnel: ["run: " "pre-run: "] -> w240
                frame False {
                }
                frame True {
                }
              }
              n254 = property on="Status Out" class="Str"("Value"=w240) -> ()  [unwired: 2 in, 2 out]
            }
            frame #1 {
              n255 = property on="Status Out" class="Str"() -> ("Value"=w251:string)  [unwired: 2 in, 2 out]
              n256 = property on="Al?" class="Bool (strict)"() -> ("Value"=w252:bool)  [unwired: 2 in, 2 out]
              n257 = property on="Run Al" class="Bool (strict)"() -> ("Value"=w244:bool)  [unwired: 2 in, 2 out]
              n258 = property on="Prep Al" class="Bool (strict)"() -> ("Value"=w246:bool)  [unwired: 2 in, 2 out]
              n259 = call "flow_strings.vi"("string in"=w251, "is first in?"=TRUE, "use source?"=w252, "name"="Al", "run source?"=w244, "prep source?"=w246, "is prep?"=w245) -> ("string out"=w250:string, "is first out?"=w249:bool)
              n260 = property on="Status Out" class="Str"("Value"=w250) -> ()  [unwired: 2 in, 2 out]
              n261 = property on="first" class="Bool (strict)"("Value"=w249) -> ()  [unwired: 2 in, 2 out]
            }
            frame #2 {
              n262 = property on="first" class="Bool (strict)"() -> ("Value"=w257:bool)  [unwired: 2 in, 2 out]
              n263 = property on="Status Out" class="Str"() -> ("Value"=w260:string)  [unwired: 2 in, 2 out]
              n264 = property on="Ga?" class="Bool (strict)"() -> ("Value"=w258:bool)  [unwired: 2 in, 2 out]
              n265 = property on="Run Ga" class="Bool (strict)"() -> ("Value"=w253:bool)  [unwired: 2 in, 2 out]
              n266 = property on="Prep Ga" class="Bool (strict)"() -> ("Value"=w255:bool)  [unwired: 2 in, 2 out]
              n267 = call "flow_strings.vi"("string in"=w260, "is first in?"=w257, "use source?"=w258, "name"="Ga", "run source?"=w253, "prep source?"=w255, "is prep?"=w254) -> ("string out"=w261:string, "is first out?"=w256:bool)
              n268 = property on="Status Out" class="Str"("Value"=w261) -> ()  [unwired: 2 in, 2 out]
              n269 = property on="first" class="Bool (strict)"("Value"=w256) -> ()  [unwired: 2 in, 2 out]
            }
            frame #3 {
              n270 = property on="first" class="Bool (strict)"() -> ("Value"=w267:bool)  [unwired: 2 in, 2 out]
              n271 = property on="Status Out" class="Str"() -> ("Value"=w269:string)  [unwired: 2 in, 2 out]
              n272 = property on="In?" class="Bool (strict)"() -> ("Value"=w270:bool)  [unwired: 2 in, 2 out]
              n273 = property on="Run In" class="Bool (strict)"() -> ("Value"=w262:bool)  [unwired: 2 in, 2 out]
              n274 = property on="Prep In" class="Bool (strict)"() -> ("Value"=w264:bool)  [unwired: 2 in, 2 out]
              n275 = call "flow_strings.vi"("string in"=w269, "is first in?"=w267, "use source?"=w270, "name"="In", "run source?"=w262, "prep source?"=w264, "is prep?"=w263) -> ("string out"=w266:string, "is first out?"=w265:bool)
              n276 = property on="Status Out" class="Str"("Value"=w266) -> ()  [unwired: 2 in, 2 out]
              n277 = property on="first" class="Bool (strict)"("Value"=w265) -> ()  [unwired: 2 in, 2 out]
            }
            frame #4 {
              n278 = property on="first" class="Bool (strict)"() -> ("Value"=w275:bool)  [unwired: 2 in, 2 out]
              n279 = property on="Status Out" class="Str"() -> ("Value"=w277:string)  [unwired: 2 in, 2 out]
              n280 = property on="PH3?" class="Bool (strict)"() -> ("Value"=w278:bool)  [unwired: 2 in, 2 out]
              n281 = property on="Run P" class="Bool (strict)"() -> ("Value"=w271:bool)  [unwired: 2 in, 2 out]
              n282 = property on="Prep P" class="Bool (strict)"() -> ("Value"=w273:bool)  [unwired: 2 in, 2 out]
              n283 = call "flow_strings.vi"("string in"=w277, "is first in?"=w275, "use source?"=w278, "name"="P", "run source?"=w271, "prep source?"=w273, "is prep?"=w272) -> ("string out"=w276:string, "is first out?"=w274:bool)
              n284 = property on="Status Out" class="Str"("Value"=w276) -> ()  [unwired: 2 in, 2 out]
              n285 = property on="first" class="Bool (strict)"("Value"=w274) -> ()  [unwired: 2 in, 2 out]
            }
            frame #5 {
              n286 = property on="first" class="Bool (strict)"() -> ("Value"=w284:bool)  [unwired: 2 in, 2 out]
              n287 = property on="Status Out" class="Str"() -> ("Value"=w286:string)  [unwired: 2 in, 2 out]
              n288 = property on="AsH3?" class="Bool (strict)"() -> ("Value"=w287:bool)  [unwired: 2 in, 2 out]
              n289 = property on="Run As" class="Bool (strict)"() -> ("Value"=w280:bool)  [unwired: 2 in, 2 out]
              n290 = property on="Prep As" class="Bool (strict)"() -> ("Value"=w282:bool)  [unwired: 2 in, 2 out]
              n291 = call "flow_strings.vi"("string in"=w286, "is first in?"=w284, "use source?"=w287, "name"="As", "run source?"=w280, "prep source?"=w282, "is prep?"=w281) -> ("string out"=w283:string, "is first out?"=w285:bool)
              n292 = property on="Status Out" class="Str"("Value"=w283) -> ()  [unwired: 2 in, 2 out]
              n293 = property on="first" class="Bool (strict)"("Value"=w285) -> ()  [unwired: 2 in, 2 out]
            }
          }
        }
        frame #3 {
          n294 = local read "run started"() -> (w294:bool)
          n295 = local read "prep_done"() -> (w292:bool)
          n296 = Not(x=w294) -> (.not. x?=w295:bool)
          n297 = And(x=w292, y=w295) -> (x .and. y?=w293:bool)
          n298 = stacked-sequence {
            tunnel: w293 -> [w299]
            tunnel: w291 -> [w298]
            tunnel: w290 -> [w297]
            tunnel: [w296] -> w289
            frame #0 {
              n299 = case shown="True" w299 {
                tunnel: w298 -> [_ w303]
                tunnel: w297 -> [w300 w302]
                tunnel: [w300 w301] -> w296
                frame False {
                }
                frame True {
                  n300 = stacked-sequence {
                    tunnel: w303 -> [w304 w311 w321 w328 w335 _]
                    tunnel: w302 -> [_ _ _ _ _ w343]
                    tunnel: [_ _ _ _ _ w342] -> w301
                    frame #0 {
                      n301 = case shown="False" w304 {
                        frame False {
                          n302 = property on="Al?" class="Bool (strict)"() -> ("Value"=w305:bool)  [unwired: 2 in, 2 out]
                          n303 = case shown="True" w305 {
                            frame False {
                              w306 = FALSE ("Al Active")
                              n304 = call "set_Al.vi"("Aluminum Flow"=0.0, "Al Remote"=w306, "Al Run"=w306, "Al Bubbler"=w306, "Al Active"=w306) -> ()  [unwired: 5 out]
                            }
                            frame True {
                              w310 = TRUE ("Al Active")
                              n305 = property on="Al Flow" class="DigNum (strict)"() -> ("Value"=w309:dbl)  [unwired: 2 in, 2 out]
                              n306 = property on="Run Al" class="Bool (strict)"() -> ("Value"=w308:bool)  [unwired: 2 in, 2 out]
                              n307 = call "set_Al.vi"("Aluminum Flow"=w309, "Al Run"=w308, "Al Bubbler"=w310, "Al Active"=w310) -> ()  [unwired: 1 in, 5 out]
                            }
                          }
                        }
                        frame True {
                        }
                      }
                    }
                    frame #1 {
                      n308 = case shown="False" w311 {
                        frame False {
                          n309 = property on="Ga?" class="Bool (strict)"() -> ("Value"=w312:bool)  [unwired: 2 in, 2 out]
                          n310 = case shown="True" w312 {
                            frame False {
                              w314 = FALSE ("Ga Active")
                              w313 = 0.0 ("Ga Flow 1")
                              n311 = call "set_Ga.vi"("Ga Active"=w314, "Ga Flow 3"=w313, "Ga Flow 2"=w313, "Ga Flow 1"=w313, "Ga Bubbler"=w314, "Ga H2 Dilute"=w314, "Ga Run"=w314, "Ga Remote"=w314) -> ()  [unwired: 8 out]
                            }
                            frame True {
                              w318 = TRUE ("Ga Active")
                              n312 = property on="Ga Dilution" class="Bool (strict)"() -> ("Value"=w317:bool)  [unwired: 2 in, 2 out]
                              n313 = property on="GAMFC3 val" class="DigNum (strict)"() -> ("Value"=w316:dbl)  [unwired: 2 in, 2 out]
                              n314 = property on="Run Ga" class="Bool (strict)"() -> ("Value"=w319:bool)  [unwired: 2 in, 2 out]
                              n315 = property on="GAMFC2 val" class="DigNum (strict)"() -> ("Value"=w320:dbl)  [unwired: 2 in, 2 out]
                              n316 = property on="GAMFC1 val" class="DigNum (strict)"() -> ("Value"=w315:dbl)  [unwired: 2 in, 2 out]
                              n317 = call "set_Ga.vi"("Ga Active"=w318, "Ga Flow 3"=w316, "Ga Flow 2"=w320, "Ga Flow 1"=w315, "Ga Bubbler"=w318, "Ga H2 Dilute"=w317, "Ga Run"=w319, "Ga Remote"=w318) -> ()  [unwired: 8 in]
                            }
                          }
                        }
                        frame True {
                        }
                      }
                    }
                    frame #2 {
                      n318 = case shown="False" w321 {
                        frame False {
                          n319 = property on="In?" class="Bool (strict)"() -> ("Value"=w322:bool)  [unwired: 2 in, 2 out]
                          n320 = case shown="True" w322 {
                            frame False {
                              w324 = FALSE ("In Remote")
                              n321 = call "set_In.vi"("Indium Flow"=0.0, "In Remote"=w324, "In Run"=w324, "In Bubbler"=w324, "In Active"=w324) -> ()  [unwired: 5 out]
                            }
                            frame True {
                              w327 = TRUE ("In Run")
                              n322 = property on="Run In" class="Bool (strict)"() -> ("Value"=w325:bool)  [unwired: 2 in, 2 out]
                              n323 = property on="In Flow" class="DigNum (strict)"() -> ("Value"=w326:dbl)  [unwired: 2 in, 2 out]
                              n324 = call "set_In.vi"("Indium Flow"=w326, "In Run"=w325, "In Bubbler"=w327, "In Active"=w327) -> ()  [unwired: 1 in, 5 out]
                            }
                          }
                        }
                        frame True {
                        }
                      }
                    }
                    frame #3 {
                      n325 = case shown="False" w328 {
                        frame False {
                          n326 = property on="PH3?" class="Bool (strict)"() -> ("Value"=w329:bool)  [unwired: 2 in, 2 out]
                          n327 = case shown="False" w329 {
                            frame False {
                              w330 = FALSE ("P_Gas Active")
                              n328 = call "set_P_gas.vi"("P_Gas Active"=w330, "P_Gas Flow"=0.0, "P_Gas In"=w330, "P_Gas H2 In"=w330, "P_Gas Run"=w330, "P_Gas Remote"=w330) -> ()  [unwired: 10 out]
                            }
                            frame True {
                              w334 = TRUE ("P_Gas Active")
                              n329 = property on="P Flow" class="DigNum (strict)"() -> ("Value"=w333:dbl)  [unwired: 2 in, 2 out]
                              n330 = property on="Run P" class="Bool (strict)"() -> ("Value"=w332:bool)  [unwired: 2 in, 2 out]
                              n331 = call "set_P_gas.vi"("P_Gas Active"=w334, "P_Gas Flow"=w333, "P_Gas In"=w334, "P_Gas Run"=w332) -> ()  [unwired: 2 in, 10 out]
                            }
                          }
                        }
                        frame True {
                        }
                      }
                    }
                    frame #4 {
                      n332 = case shown="False" w335 {
                        frame False {
                          n333 = property on="AsH3?" class="Bool (strict)"() -> ("Value"=w336:bool)  [unwired: 2 in, 2 out]
                          n334 = case shown="True" w336 {
                            frame False {
                              w337 = FALSE ("As_Gas Active")
                              n335 = call "set_As_gas.vi"("As_Gas Active"=w337, "As_Gas Flow"=0.0, "As_Gas In"=w337, "As_Gas H2"=w337, "As_Gas Run"=w337, "As_Gas Remote"=w337) -> ()  [unwired: 10 in]
                            }
                            frame True {
                              w340 = TRUE ("As_Gas Active")
                              n336 = property on="Run As" class="Bool (strict)"() -> ("Value"=w339:bool)  [unwired: 2 in, 2 out]
                              n337 = property on="AsH3 Flow" class="DigNum (strict)"() -> ("Value"=w341:dbl)  [unwired: 2 in, 2 out]
                              n338 = call "set_As_gas.vi"("As_Gas Active"=w340, "As_Gas Flow"=w341, "As_Gas In"=w340, "As_Gas Run"=w339) -> ()  [unwired: 12 in]
                            }
                          }
                        }
                        frame True {
                        }
                      }
                    }
                    frame #5 {
                      n339 = call "Set_Argument.vi"("Enable"=TRUE, "Argument"="run_started", "Argument List In"=w343) -> ("Argument List Out"=w342:string[])
                    }
                  }
                }
              }
            }
          }
        }
      }
    }
    frame "End" {
    }
    frame "Idle" {
    }
  }
  "Argument List Out" <- w10
